vi "TSM Relay Per-Site to Per-Instrument Data.vi"(0 "SSC Relay":T1[](array[typedef]), 5 "TSM Site Numbers":i32[](array[numeric]), 7 "Completed Relay Operations":T2[](array[typedef]) {"Desired State" items=["Open Relay"=20, "Close Relay"=21]}, 9 "Selection":enum16{"Desired State", "Relay Operated?"}(ring)) -> (4 "Per-Instrument Per-Relay Data":i32[][](array[numeric]))   [LabVIEW 2019]
doc: "This VI takes either the Desired State or Relay Operated? information from the Completed Relay Operations cluster and orders it to be Per-Instrument Per-Relay, which is the format required by the TSM Publish VI."
uses:
  TSM Relay Completed Operations.ctl
  <instrlib>/niSwitch/niSwitch.llb/niSwitch Relay Action.ctl
  SSC/SSC Relay.ctl
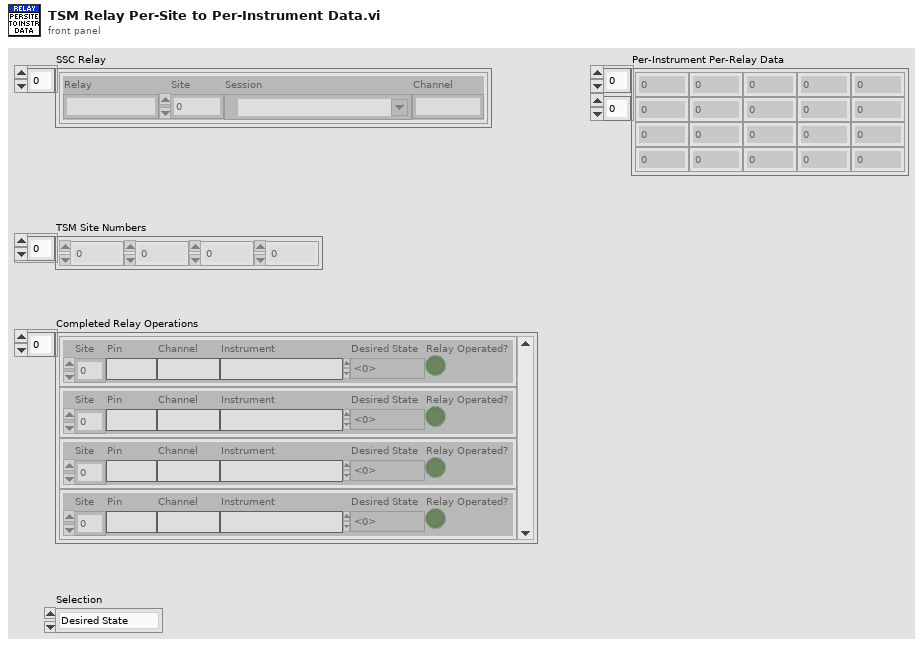
[diagram p1: front panel]
types:
  T1 = typedef "SSC Relay.ctl" = cluster{"Relay":string, "Site":i32, "Session":refnum<k15>, "Channel":string}
  T2 = typedef "TSM Relay Completed Operations.ctl" = cluster{"Site":i32, "Pin":string, "Channel":string, "Instrument":string, "Desired State":T3, "Relay Operated?":bool}
  T3 = typedef "niSwitch Relay Action.ctl" = i32
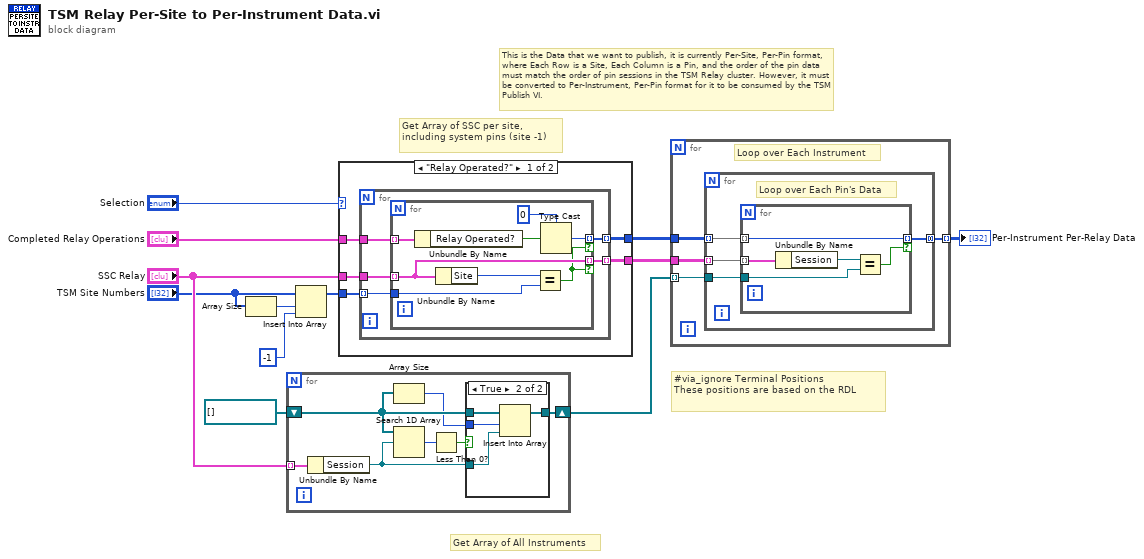
[diagram p0: block diagram]
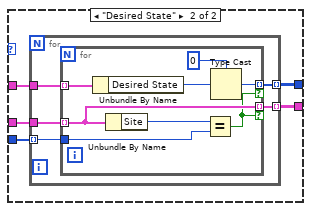
[diagram p2: hidden frame]
diagram:
  # "#via_ignore Terminal Positions\nThese positions are based on the RDL"
  # "Get Array of SSC per site, including system pins (site -1)"
  # "Get Array of All Instruments"
  # "This is the Data that we want to publish, it is currently Per-Site, Per-Pin format, where Each Row is a Site, Each Column is a Pin, and the order of the pin data must match the order of pin sessions in the TSM Relay cluster. However, it must be converted to Per-Instrument, Per-Pin format for it to be consumed by the TSM Publish VI."
  n1 = Array Size(array="TSM Site Numbers") -> (size(s)=w9:i32)
  n2 = for {
    tunnel: "SSC Relay" -> [w19] mode=indexing
    shift-right: [w18] -> w10
    shift-left: refnum<k15>[] [] -> [w14]
    n3 = Unbundle By Name(w19) -> ("Session"=w17:refnum<k15>)
    n4 = Array Size(array=w14) -> (size(s)=w13:i32)
    n5 = Search 1D Array(1D array=w14, element=w17) -> (index of element=w16:i32)  [unwired: 1 in]
    n6 = Less Than 0?(x=w16) -> (x < 0?=w15:bool)
    n7 = case shown="True" w15 {
      tunnel: w17 -> [_ w24]
      tunnel: w14 -> [w20 w23]
      tunnel: [w20 w22] -> w18
      tunnel: w13 -> [_ w21]
      frame False {
      }
      frame True {
        n8 = Insert Into Array(array=w23, index=w21, new element=w24) -> (w22:refnum<k15>[])
      }
    }
  }
  n9 = Insert Into Array(array="TSM Site Numbers", index=w9, new element=-1) -> (w7:i32[])
  n10 = case shown="\"Relay Operated?\"" "Selection" {
    tunnel: [w29 w47] -> w8
    tunnel: w7 -> [w28 w46]
    tunnel: "Completed Relay Operations" -> [w27 w45]
    tunnel: [w26 w44] -> w4
    tunnel: "SSC Relay" -> [w25 w43]
    frame "Relay Operated?" {
      n11 = for {
        tunnel: w25 -> [w34]
        tunnel: [w33] -> w29 mode=indexing
        tunnel: w28 -> [w32] mode=indexing
        tunnel: w27 -> [w31]
        tunnel: [w30] -> w26 mode=indexing
        n12 = for {
          tunnel: w34 -> [w42] mode=indexing
          tunnel: [w42] -> w33 mode=indexing if=w37
          tunnel: w32 -> [w41]
          tunnel: w31 -> [w39] mode=indexing
          tunnel: [w36] -> w30 mode=indexing if=w37
          n13 = Unbundle By Name(w39) -> ("Relay Operated?"=w38:bool)
          n14 = Unbundle By Name(w42) -> ("Site"=w40:i32)
          n15 = Equal?(x=w40, y=w41) -> (x = y?=w37:bool)
          n16 = Type Cast(type=0 ("32bit integer"), x=w38) -> (*(type *) &x=w36:i32)
        }
      }
    }
    frame "Desired State" {
      n17 = for {
        tunnel: w43 -> [w52]
        tunnel: [w51] -> w47 mode=indexing
        tunnel: w46 -> [w50] mode=indexing
        tunnel: w45 -> [w49]
        tunnel: [w48] -> w44 mode=indexing
        n18 = for {
          tunnel: w52 -> [w60] mode=indexing
          tunnel: [w60] -> w51 mode=indexing if=w55
          tunnel: w50 -> [w59]
          tunnel: w49 -> [w57] mode=indexing
          tunnel: [w54] -> w48 mode=indexing if=w55
          n19 = Unbundle By Name(w57) -> ("Desired State"=w56:T3)
          n20 = Unbundle By Name(w60) -> ("Site"=w58:i32)
          n21 = Equal?(x=w58, y=w59) -> (x = y?=w55:bool)
          n22 = Type Cast(type=0 ("32bit integer"), x=w56) -> (*(type *) &x=w54:i32)
        }
      }
    }
  }
  n23 = for {
    tunnel: w8 -> [w64]
    tunnel: w10 -> [w63] mode=indexing
    tunnel: w4 -> [w62]
    tunnel: [w61] -> w5 mode=indexing
    # "Loop over Each Instrument"
    n24 = for {
      tunnel: w64 -> [w67] mode=indexing
      tunnel: w63 -> [w68]
      tunnel: w62 -> [w65] mode=indexing
      tunnel: [w66] -> w61 mode=concatenating
      # "Loop over Each Pin's Data"
      n25 = for {
        tunnel: w67 -> [w73] mode=indexing
        tunnel: w68 -> [w71]
        tunnel: w65 -> [w70] mode=indexing
        tunnel: [w70] -> w66 mode=indexing if=w69
        n26 = Unbundle By Name(w73) -> ("Session"=w72:refnum<k15>)
        n27 = Equal?(x=w72, y=w71) -> (x = y?=w69:bool)
      }
    }
  }
  "Per-Instrument Per-Relay Data" <- w5
